vi "Get Attribute.vi"(8 "error in":errorcluster, 10 "Attribute":string, 11 "Config from EXCEL Table in":refnum<class "Config from Excel Table.lvclass">) -> (0 "error out":errorcluster, 2 "Value":variant, 3 "Config from EXCEL Table out":refnum<class "Config from Excel Table.lvclass">)   [LabVIEW 2025, in "Config from Excel Table.lvclass"]
uses:
  Config from Excel Table.lvclass
  Config from Excel Table.lvclass/Config from Excel Table.ctl
  Open-Xml-LabVIEW/Source/Open Xml.lvlib
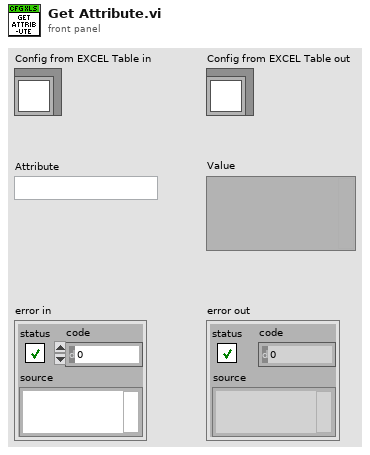
[diagram p1: front panel]
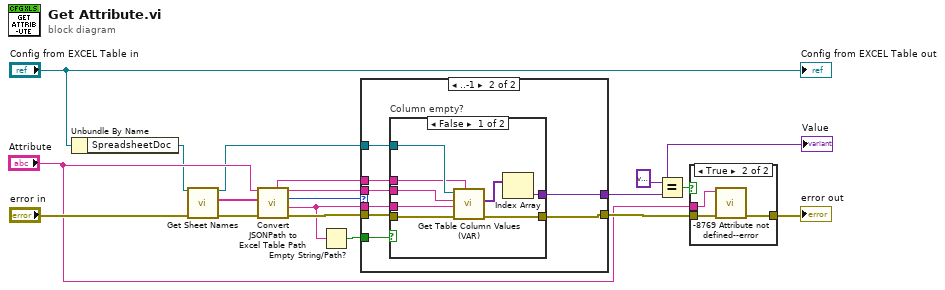
[diagram p0: block diagram]
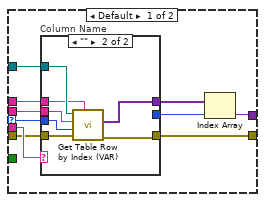
[diagram p2: hidden frame]
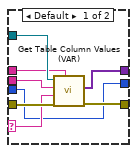
[diagram p3: hidden frame]
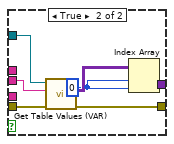
[diagram p4: hidden frame]
diagram:
  n1 = Unbundle By Name("Config from EXCEL Table in") -> ("SpreadsheetDoc"=w3:refnum<k24>)
  n2 = call "Get Sheet Names.vi"("error in"="error in", "SpreadsheetDoc in"=w3) -> ("error out"=w4:errorcluster, "Sheet Names"=w1:string[], "SpreadsheetDoc out"=w2:refnum<k24>)  [unwired: 7 in]
  n3 = call "Convert JSONPath to Excel Table Path.vi"("error in"=w4, "Sheet Names"=w1, "JSONPath"="Attribute") -> ("error out"=w16:errorcluster, "Column"=w7:string, "Row"=w6:i32, "Table Name"=w17:string, "Sheet Name"=w5:string)  [unwired: 4 in]
  n4 = Empty String/Path?(string/path=w7) -> (empty?=w18:bool)
  n5 = case shown="..-1" w6 {
    selector: w6 -> [w25 _]
    tunnel: w18 -> [_ w51]
    tunnel: w2 -> [w23 w50]
    tunnel: w17 -> [w24 w49]
    tunnel: w16 -> [w26 w48]
    tunnel: [w27 w47] -> w13
    tunnel: [w21 w46] -> w10
    tunnel: w7 -> [w28 w45]
    tunnel: w5 -> [w19 w44]
    frame Default {
      n6 = case "Column Name" shown="\"\"" w28 {
        selector: w28 -> [w34 _]
        tunnel: [w35 w39] -> w27
        tunnel: w26 -> [w36 w43]
        tunnel: w25 -> [w30 w42]
        tunnel: w24 -> [w33 w41]
        tunnel: w23 -> [w32 w40]
        tunnel: [w31 w38] -> w22
        tunnel: [w30 _] -> w20
        tunnel: w19 -> [w29 w37]
        frame Default {
          n7 = call "Get Table Column Values (VAR).vi"("Sheet Name in"=w29, "error in"=w36, "Column Name"=w34, "Table Name"=w33, "SpreadsheetDoc in"=w32) -> ("error out"=w35:errorcluster, "Column Values"=w31:variant[])  [unwired: 4 in, 1 out]
        }
        frame "" {
          n8 = call "Get Table Row by Index (VAR).vi"("Sheet Name"=w37, "error in"=w43, "Row Index"=w42, "Table Name"=w41, "SpreadsheetDoc in"=w40) -> ("error out"=w39:errorcluster, "Rows"=w38:variant[])  [unwired: 4 in, 1 out]
        }
      }
      n9 = Index Array(array=w22, index=w20) -> (element=w21:variant)
    }
    frame ..-1 {
      n10 = case "Column empty?" shown="False" w51 {
        tunnel: w48 -> [w59 w66]
        tunnel: [w58 w61] -> w47
        tunnel: w50 -> [w57 w65]
        tunnel: w49 -> [w56 w64]
        tunnel: w45 -> [w55 _]
        tunnel: [w53 w60] -> w46
        tunnel: w44 -> [w52 _]
        frame False {
          n11 = call "Get Table Column Values (VAR).vi"("Sheet Name in"=w52, "error in"=w59, "Column Name"=w55, "Table Name"=w56, "SpreadsheetDoc in"=w57) -> ("error out"=w58:errorcluster, "Column Values"=w54:variant[])  [unwired: 4 in, 1 out]
          n12 = Index Array(array=w54) -> (element=w53:variant)  [unwired: 1 in]
        }
        frame True {
          w62 = 0 ("index (col)")
          n13 = call "Get Table Values (VAR).vi"("error in"=w66, "Table Name"=w64, "SpreadsheetDoc in"=w65) -> ("error out"=w61:errorcluster, "Table Values"=w63:variant[][])  [unwired: 6 in, 1 out]
          n14 = Index Array(array=w63, index (row)=w62, index (col)=w62) -> (element=w60:variant)
        }
      }
    }
  }
  "Value" <- w10
  n15 = Equal?(x=variant, y=w10) -> (x = y?=w11:bool)
  n16 = case shown="True" w11 {
    tunnel: w13 -> [w67 w70]
    tunnel: [w67 w69] -> w12
    tunnel: "Attribute" -> [_ w68]
    frame False {
    }
    frame True {
      n17 = call "-8769 Attribute not defined--error.vi"("error in"=w70, "Argument"=w68) -> ("error out"=w69:errorcluster)  [unwired: 8 in, 1 out]
    }
  }
  "error out" <- w12
  "Config from EXCEL Table out" <- "Config from EXCEL Table in"
